vi "START TRANSFER ITEMS.vi"(10 "USER/ITEM DATA TRANSFER IN":T2(array[cluster]), 11 "REFERENCES":T3) -> (2 "DATA OUT":T1[](array[typedef]), 3 "BYU ID #":string)   [LabVIEW 2019]
uses:
  Controls/References Cluster.ctl
  <vilib>/userDefined/High Color/IMAQdx.ctl
  Controls/Custom Calendar/Custom Calendar.xctl
  Controls/Table Data Types/Inventory Data Type.ctl
  <vilib>/Utility/miscctls.llb/LVRowAndColumnTypeDef.ctl
  <vilib>/addons/database/Connection.llb/DB Tools Open Connec (String).vi
  <vilib>/addons/database/_DB Variant To Data/Database Variant To Data.xnode
  <vilib>/addons/database/NI_Database_API.lvlib
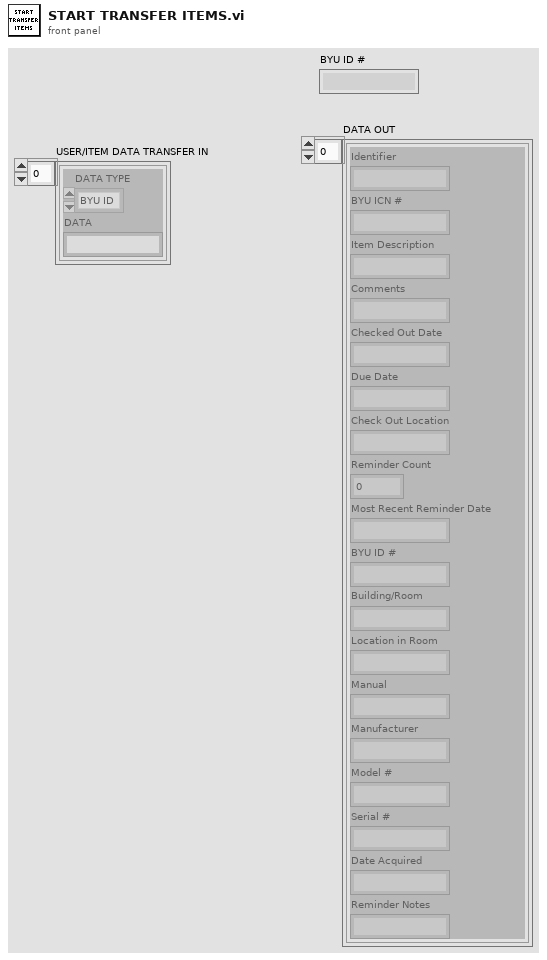
[diagram p1: front panel]
types:
  T1 = typedef "Inventory Data Type.ctl" = cluster{"Identifier":string, "BYU ICN #":string, "Item Description":string, "Comments":string, "Checked Out Date":string, "Due Date":string, "Check Out Location":string, "Reminder Count":i32, "Most Recent Reminder Date":string, "BYU ID #":string, "Building/Room":string, "Location in Room":string, "Manual":string, "Manufacturer":string, "Model #":string, "Serial #":string, "Date Acquired":string, "Reminder Notes":string}
  T2 = cluster{"DATA TYPE":enum16{"BYU ID", "ME#/IDENTIFIER", "BYU ICN"}, "DATA":string}[]
  T3 = typedef "References Cluster.ctl" = cluster{"MAIN PAGES":refnum<vi>, "ADD/EDIT ITEM REFERENCES":cluster{"Identifier":refnum<vi>, "BYU ICN #":refnum<vi>, "Item Description":refnum<vi>, "Comments":refnum<vi>, "Checked Out Date":refnum<vi>, "Due Date":refnum<vi>, "Check Out Location":refnum<vi>, "Reminder Count":refnum<vi>, "Most Recent Reminder Date":refnum<vi>, "BYU ID #":refnum<vi>, "Building/Room":refnum<vi>, "Location in Room":refnum<vi>, "Manual":refnum<vi>, "Manufacturer":refnum<vi>, "Model #":refnum<vi>, "Serial #":refnum<vi>, "Date Acquired":refnum<vi>, "ADD/EDIT ITEM LABEL":refnum<vi>, "ARCHIVE ITEM":refnum<vi>, "Archive Item Inputs":refnum<vi>, "Reminder Notes":refnum<vi>}, "ADD/EDIT USER REFERENCES":cluster{"BYU ID # (##-###-####)":refnum<vi>, "First Name":refnum<vi>, "Last Name":refnum<vi>, "Phone Number (###-###-####)":refnum<vi>, "Email":refnum<vi>, "Department":refnum<vi>, "Graduation Status":refnum<vi>, "Anticipated Graduation Year":refnum<vi>, "Credit Score":refnum<vi>, "Date Added":refnum<vi>, "Graduation Clearance Date":refnum<vi>, "Picture File Name":refnum<vi>, "ADD/EDIT USER LABEL":refnum<vi>, "Department Map":refnum<vi>, "Status Map":refnum<vi>, "Anticipated Graduation Year Map":refnum<vi>, "User Agreement":refnum<vi>, "User Comments":refnum<vi>, "Camera":refnum<vi>}, "RETURN ITEM REFERENCES":cluster{"Item or Person:":refnum<vi>, "Search Return Results":refnum<vi>, "What are you searching for?":refnum<vi>}, "SEARCH DATABASE REFERENCES":cluster{"What to Search For:":refnum<vi>, "Where to Search":refnum<vi>, "Column to Search In":refnum<vi>, "Column to Sort By":refnum<vi>, "Search Database Results":refnum<vi>, "Inventory Column Selector":refnum<vi>, "User Column Selector":refnum<vi>, "Inventory Archive Column Selector":refnum<vi>, "User Archive Column Selector":refnum<vi>, "Sales Tracking Column Selector":refnum<vi>, "Checked In Archive Column Selector":refnum<vi>, "Restore User":refnum<vi>, "Date Range":refnum<vi>, "Dates Less Than":refnum<vi>, "Dates Greater Than":refnum<vi>, "Search Print Receipt":refnum<vi>, "Edit Sale Description":refnum<vi>}, "USER ITEMS REFERENCES":cluster{"USER'S INFORMATION":refnum<vi>, "User's Checked Out Items":refnum<vi>, "User Info Comments":refnum<vi>, "SEE USER INFO COMMENTS":refnum<vi>}, "EDIT ITEMS REFERENCES":cluster{"New Check Out Location":refnum<vi>, "Items to Edit":refnum<vi>, "Edit Items Due Date":refnum<vi>, "New Reminder Notes":refnum<vi>, "New Item Description":refnum<vi>}, "CHECK OUT ITEMS REFERENCES":cluster{"Enter Item:":refnum<vi>, "Check Out Items Due Date":refnum<vi>, "Check Out Location":refnum<vi>, "Items to be Checked Out":refnum<vi>, "Possible Items":refnum<vi>}, "TRANSFER ITEMS REFERENCES":cluster{"Search Parameter":refnum<vi>, "What to Match":refnum<vi>, "Matching Individuals":refnum<vi>, "Items to be Transferred":refnum<vi>}, "SETTINGS REFERENCES":cluster{"PSC Database Settings":refnum<vi>, "PSC Sales Item Spreadsheet":refnum<vi>}, "PSC SALES REFERENCES":cluster{"BYU ID CARD #":refnum<vi>, "Sale Description":refnum<vi>, "Scan or Enter Item Name":refnum<vi>, "Items to be Sold":refnum<vi>, "Grand Total":refnum<vi>, "Item List":refnum<vi>}}
  T4 = typedef "LVRowAndColumnTypeDef.ctl" = cluster{"Row":i32, "Column":i32}
  T5 = enum32{"IDLE", "ADD/EDIT USER", "ADD/EDIT ITEM", "RETURN ITEMS", "SEARCH DATABASE", "USER ITEMS", "CHECK OUT ITEMS", "EDIT ITEMS", "TRANSFER ITEMS", "PSC SALES", "ATRIUM", "INVENTORY TRACKING", "SETTINGS"}
  T6 = typedef "NI_Database_API.lvlib/Conn ObjectReference.ctl" = refnum<k1>
  T7 = cluster{"Search Parameter":refnum<vi>, "What to Match":refnum<vi>, "Matching Individuals":refnum<vi>, "Items to be Transferred":refnum<vi>}
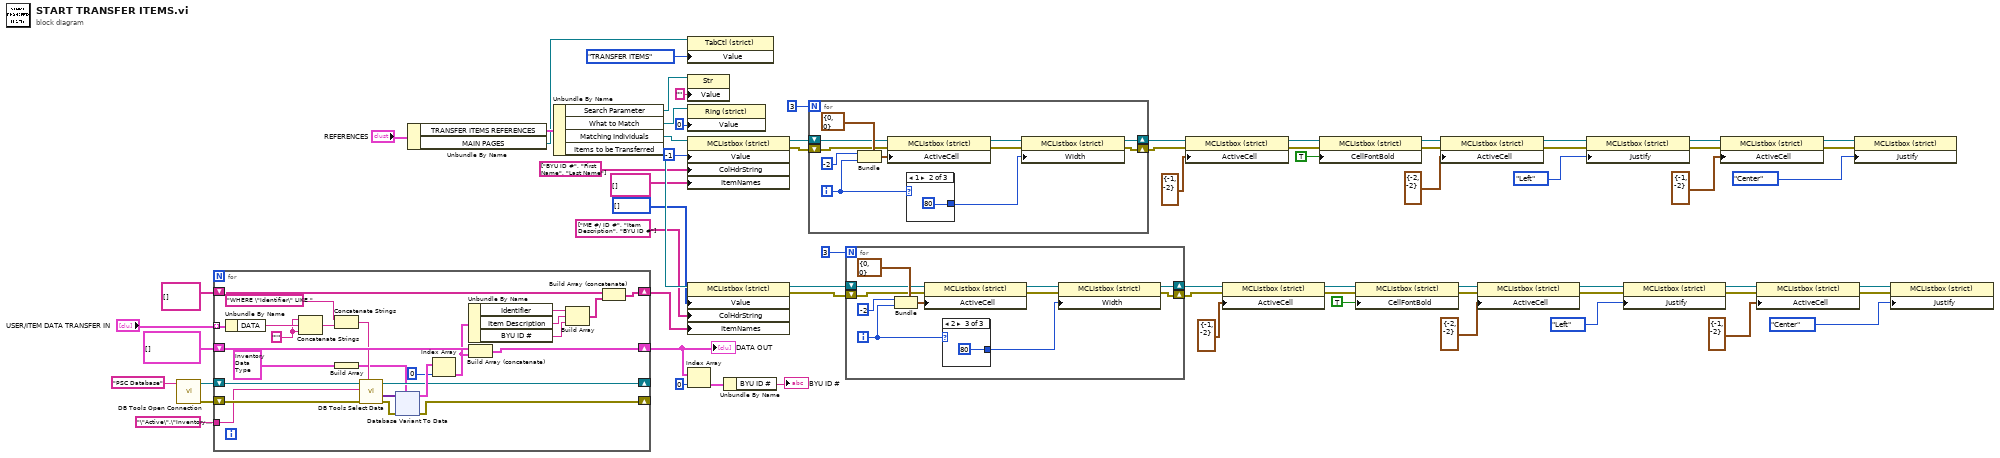
[diagram p0: block diagram]
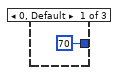
[diagram p2: hidden frame]
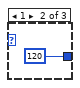
[diagram p3: hidden frame]
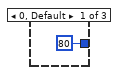
[diagram p4: hidden frame]
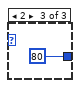
[diagram p5: hidden frame]
diagram:
  n1 = call-poly <vilib>:"DB Tools Open Connection.vi"("connection information"="PSC Database" ("Value")) -> ("error out"=w56:errorcluster, "connection reference"=w57:T6)  [unwired: 7 in]
  n2 = for {
    tunnel: "USER/ITEM DATA TRANSFER IN" -> [w93] mode=indexing
    shift-right: [w87] -> _
    shift-left: w57 -> [w95]
    shift-right: [w86] -> _
    shift-left: w56 -> [w94]
    shift-right: [w85] -> w51
    shift-left: T1[] [] ("DATA OUT") -> [w84]
    tunnel: "\"Active\".\"Inventory\"" ("Value") -> [w92]
    shift-right: [w75] -> w52
    shift-left: string[][] [] ("Item Names") -> [w77]
    w70 = "'"
    n3 = Unbundle By Name(w93) -> ("DATA"=w71:string)
    n4 = Concatenate Strings(w70, w71, w70) -> (w72:string)
    n5 = Concatenate Strings("WHERE \"Identifier\" LIKE " ("Value"), w72) -> (w82:string)
    n6 = Build Array(T1 {"Identifier"="", "BYU ICN #"="", "Item Description"="", "Comments"="", "Checked Out Date"="", "Due Date"="", "Check Out Location"="", "Reminder Count"=0, "Most Recent Reminder Date"="", "BYU ID #"="", "Building/Room"="", "Location in Room"="", "Manual"="", "Manufacturer"="", "Model #"="", "Serial #"="", "Date Acquired"="", "Reminder Notes"=""} ("Cluster")) -> (w73:T1[])
    n7 = call <vilib>:"DB Tools Select Data.vi"("condition"=w82, "error in (no error)"=w94, "table"=w92, "connection reference"=w95) -> ("error out"=w90:errorcluster, "data"=w91:variant[][], "connection reference out"=w87:T6)  [unwired: 2 in]
    n8 = xnode "Database Variant To Data"("database variant"=w91, "error in (no error)"=w90, "type"=w73) -> ("data"=w89:T1[], "error out"=w86:errorcluster)
    n9 = Index Array(array=w89, index=0) -> (element=w81:T1)
    n10 = Unbundle By Name(w81) -> ("Identifier"=w80:string, "Item Description"=w78:string, "BYU ID #"=w79:string)
    n11 = Build Array (concatenate)(w84, w81) -> (w85:T1[])
    n12 = Build Array(w80, w78, w79) -> (w76:string[])
    n13 = Build Array (concatenate)(w77, w76) -> (w75:string[][])
  }
  "DATA OUT" <- w51
  n14 = Unbundle By Name("REFERENCES") -> ("TRANSFER ITEMS REFERENCES"=w68:T7, "MAIN PAGES"=w46:refnum<vi>)
  n15 = Unbundle By Name(w68) -> ("Search Parameter"=w67:refnum<vi>, "What to Match"=w65:refnum<vi>, "Matching Individuals"=w63:refnum<vi>, "Items to be Transferred"=w62:refnum<vi>)
  n16 = property class="TabCtl (strict)"(reference=w46, "Value"=T5."TRANSFER ITEMS") -> ()  [unwired: 1 in, 2 out]
  n17 = property class="Str"(reference=w67, "Value"="") -> ()  [unwired: 1 in, 2 out]
  n18 = property class="Ring (strict)"(reference=w65, "Value"=u16 0) -> ()  [unwired: 1 in, 2 out]
  n19 = property class="MCListbox (strict)"(reference=w63, "Value"=-1, "ColHdrString"=string[] ["BYU ID #", "First Name", "Last Name"] ("Column Header Strings[]"), "ItemNames"=string[][] [] ("Item Names")) -> (reference out=w23:refnum<vi>, error out=w22:errorcluster)  [unwired: 1 in]
  n20 = property class="MCListbox (strict)"(reference=w62, "Value"=i32[] [], "ColHdrString"=string[] ["ME #/ ID #", "Item Description", "BYU ID #"] ("Column Header Strings[]"), "ItemNames"=w52) -> (reference out=w2:refnum<vi>, error out=w1:errorcluster)  [unwired: 1 in]
  n21 = Index Array(array=w51, index=0) -> (element=w49:T1)
  n22 = Unbundle By Name(w49) -> ("BYU ID #"=→"BYU ID #":string)
  n23 = for {
    N: 3 -> [_]
    shift-right: [w674] -> w24
    shift-left: w23 -> [w671]
    shift-right: [w673] -> w25
    shift-left: w22 -> [w670]
    i -> [w667]
    n24 = Bundle(cluster=T4 {"Row"=0, "Column"=0} ("Active Cell:Active Cell"), "Row"=-2, "Column"=w667) -> (w669:T4)
    n25 = property class="MCListbox (strict)"(reference=w671, error in=w670, "ActiveCell"=w669) -> (reference out=w665:refnum<vi>, error out=w664:errorcluster)
    n26 = case shown="1" w667 {
      tunnel: [u32 80 ("Active Cell:Cell Size:Width") u32 80 ("Active Cell:Cell Size:Width") u32 80 ("Active Cell:Cell Size:Width")] -> w666
      frame 0, Default {
      }
      frame 1 {
      }
      frame 2 {
      }
    }
    n27 = property class="MCListbox (strict)"(reference=w665, error in=w664, "Width"=w666) -> (reference out=w674:refnum<vi>, error out=w673:errorcluster)
  }
  n28 = for {
    N: 3 -> [_]
    shift-right: [w688] -> w3
    shift-left: w2 -> [w685]
    shift-right: [w687] -> w4
    shift-left: w1 -> [w684]
    i -> [w681]
    n29 = Bundle(cluster=T4 {"Row"=0, "Column"=0} ("Active Cell:Active Cell"), "Row"=-2, "Column"=w681) -> (w683:T4)
    n30 = property class="MCListbox (strict)"(reference=w685, error in=w684, "ActiveCell"=w683) -> (reference out=w679:refnum<vi>, error out=w678:errorcluster)
    n31 = case shown="2" w681 {
      tunnel: [u32 70 ("Active Cell:Cell Size:Width") u32 120 ("Active Cell:Cell Size:Width") u32 80 ("Active Cell:Cell Size:Width")] -> w680
      frame 0, Default {
      }
      frame 1 {
      }
      frame 2 {
      }
    }
    n32 = property class="MCListbox (strict)"(reference=w679, error in=w678, "Width"=w680) -> (reference out=w688:refnum<vi>, error out=w687:errorcluster)
  }
  n33 = property class="MCListbox (strict)"(reference=w24, error in=w25, "ActiveCell"=T4 {"Row"=-1, "Column"=-2} ("Active Cell:Active Cell")) -> (reference out=w41:refnum<vi>, error out=w40:errorcluster)
  n34 = property class="MCListbox (strict)"(reference=w3, error in=w4, "ActiveCell"=T4 {"Row"=-1, "Column"=-2} ("Active Cell:Active Cell")) -> (reference out=w20:refnum<vi>, error out=w19:errorcluster)
  n35 = property class="MCListbox (strict)"(reference=w41, error in=w40, "CellFontBold"=TRUE ("Active Cell:Cell Font:Bold")) -> (reference out=w38:refnum<vi>, error out=w37:errorcluster)
  n36 = property class="MCListbox (strict)"(reference=w20, error in=w19, "CellFontBold"=TRUE ("Active Cell:Cell Font:Bold")) -> (reference out=w17:refnum<vi>, error out=w16:errorcluster)
  n37 = property class="MCListbox (strict)"(reference=w38, error in=w37, "ActiveCell"=T4 {"Row"=-2, "Column"=-2} ("Active Cell:Active Cell")) -> (reference out=w35:refnum<vi>, error out=w34:errorcluster)
  n38 = property class="MCListbox (strict)"(reference=w17, error in=w16, "ActiveCell"=T4 {"Row"=-2, "Column"=-2} ("Active Cell:Active Cell")) -> (reference out=w14:refnum<vi>, error out=w13:errorcluster)
  n39 = property class="MCListbox (strict)"(reference=w35, error in=w34, "Justify"=enum16{"Left", "Center", "Right"}."Left" ("Active Cell:Cell Justification")) -> (reference out=w30:refnum<vi>, error out=w29:errorcluster)
  n40 = property class="MCListbox (strict)"(reference=w14, error in=w13, "Justify"=enum16{"Left", "Center", "Right"}."Left" ("Active Cell:Cell Justification")) -> (reference out=w9:refnum<vi>, error out=w8:errorcluster)
  n41 = property class="MCListbox (strict)"(reference=w30, error in=w29, "ActiveCell"=T4 {"Row"=-1, "Column"=-2} ("Active Cell:Active Cell")) -> (reference out=w31:refnum<vi>, error out=w32:errorcluster)
  n42 = property class="MCListbox (strict)"(reference=w9, error in=w8, "ActiveCell"=T4 {"Row"=-1, "Column"=-2} ("Active Cell:Active Cell")) -> (reference out=w10:refnum<vi>, error out=w11:errorcluster)
  n43 = property class="MCListbox (strict)"(reference=w31, error in=w32, "Justify"=enum16{"Left", "Center", "Right"}."Center" ("Active Cell:Cell Justification")) -> ()  [unwired: 2 out]
  n44 = property class="MCListbox (strict)"(reference=w10, error in=w11, "Justify"=enum16{"Left", "Center", "Right"}."Center" ("Active Cell:Cell Justification")) -> ()  [unwired: 2 out]
